vi "CALIBRATE 2016.vi"(0 "flow_slope_IN":dbl=51.35 format="%.2f", 1 "pressure_slope_IN":dbl=23.33 format="%.2f", 3 "DHT_Pressure Slope":dbl=1.5 format="%.2f", 4 "Descriptions":string[](array[string]), 5 "string_pot_slope_IN":dbl=1.5 format="%.2f", 6 "DHT_Pressure_Offset":dbl=1.5 format="%.2f", 7 "error in (no error)":errorcluster, 8 "Array in":refnum<k24>[](array[refnum]), 9 "Sensor Cluster":T2, 12 "Aux1_Slope In":dbl=1.5 format="%.2f", 13 "Aux3_ Slope In":dbl=1.5 format="%.2f", 16 "Aux2_Slope In":dbl=1.5 format="%.2f", 17 "Path":path=path "C:/Cascade/Data/Output Files") -> (14 "Array out":refnum<k24>[](array[refnum]), 15 "Sensor Cluster 2":T2, 19 "Output Slopes Cluster":T1={"DHT_Pressure Slope Out"=1.5, "DHT_Pressure_Offset Out"=1.5, "Aux1_Slope Out"=1.5, "Aux2_Slope Out"=1.5, "Aux3_ Slope Out"=1.5, "string_pot_slope_OUT"=1.5, "flow_slope_OUT"=51.35, "pressure_slope_OUT"=23.33} {"pressure_slope_OUT" format="%.2f"; "flow_slope_OUT" format="%.2f"; "string_pot_slope_OUT" format="%.2f"; "Aux3_ Slope Out" format="%.2f"; "Aux2_Slope Out" format="%.2f"; "Aux1_Slope Out" format="%.2f"; "DHT_Pressure_Offset Out" format="%.2f"; "DHT_Pressure Slope Out" format="%.2f"}, 20 "flow_slope_OUT":dbl=51.35 format="%.2f", 21 "pressure_slope_OUT":dbl=23.33 format="%.2f", 23 "Record Output Slopes to  Record File":path, 24 "Record Output Slopes for slopes.csv File":path, 25 "string_pot_slope_OUT":dbl=1.5 format="%.2f", 27 "error out":errorcluster)   [LabVIEW 2016]
uses:
  controls/MCC DAQ Readings.ctl
  C:/Program Files/National Instruments/LabVIEW 2016/vi.lib/ULx/ULx_LV.dll
  Program Files/National Instruments/LabVIEW 2016/vi.lib/ULx/ULx_LV.dll
  Kpro Globals.vi
panel:
  in  "Distance from APS Tip to transducer (ft)":dbl=5.2 format="%.2f"
  out "Aux3_ Slope Out":dbl=1.5 format="%.2f"
  out "Aux2_Slope Out":dbl=1.5 format="%.2f"
  out "Aux1_Slope Out":dbl=1.5 format="%.2f"
  out "DHT_Pressure_Offset Out":dbl=1.5 format="%.2f"
  out "DHT_Pressure Slope Out":dbl=1.5 format="%.2f"
  in  "all PFS":bool
  in  "Aux 3 Calibrate":bool
  in  "Aux 2 Calibrate":bool
  in  "Aux 1 Calibrate":bool
  in  "DHT":bool
  out "Loop Counter":i32
  in  "exit":bool
  in  "string_pot":bool
  in  "pressure":bool
  in  "flow":bool
  in  "start path":path=path "C:/"
  in  "all":bool
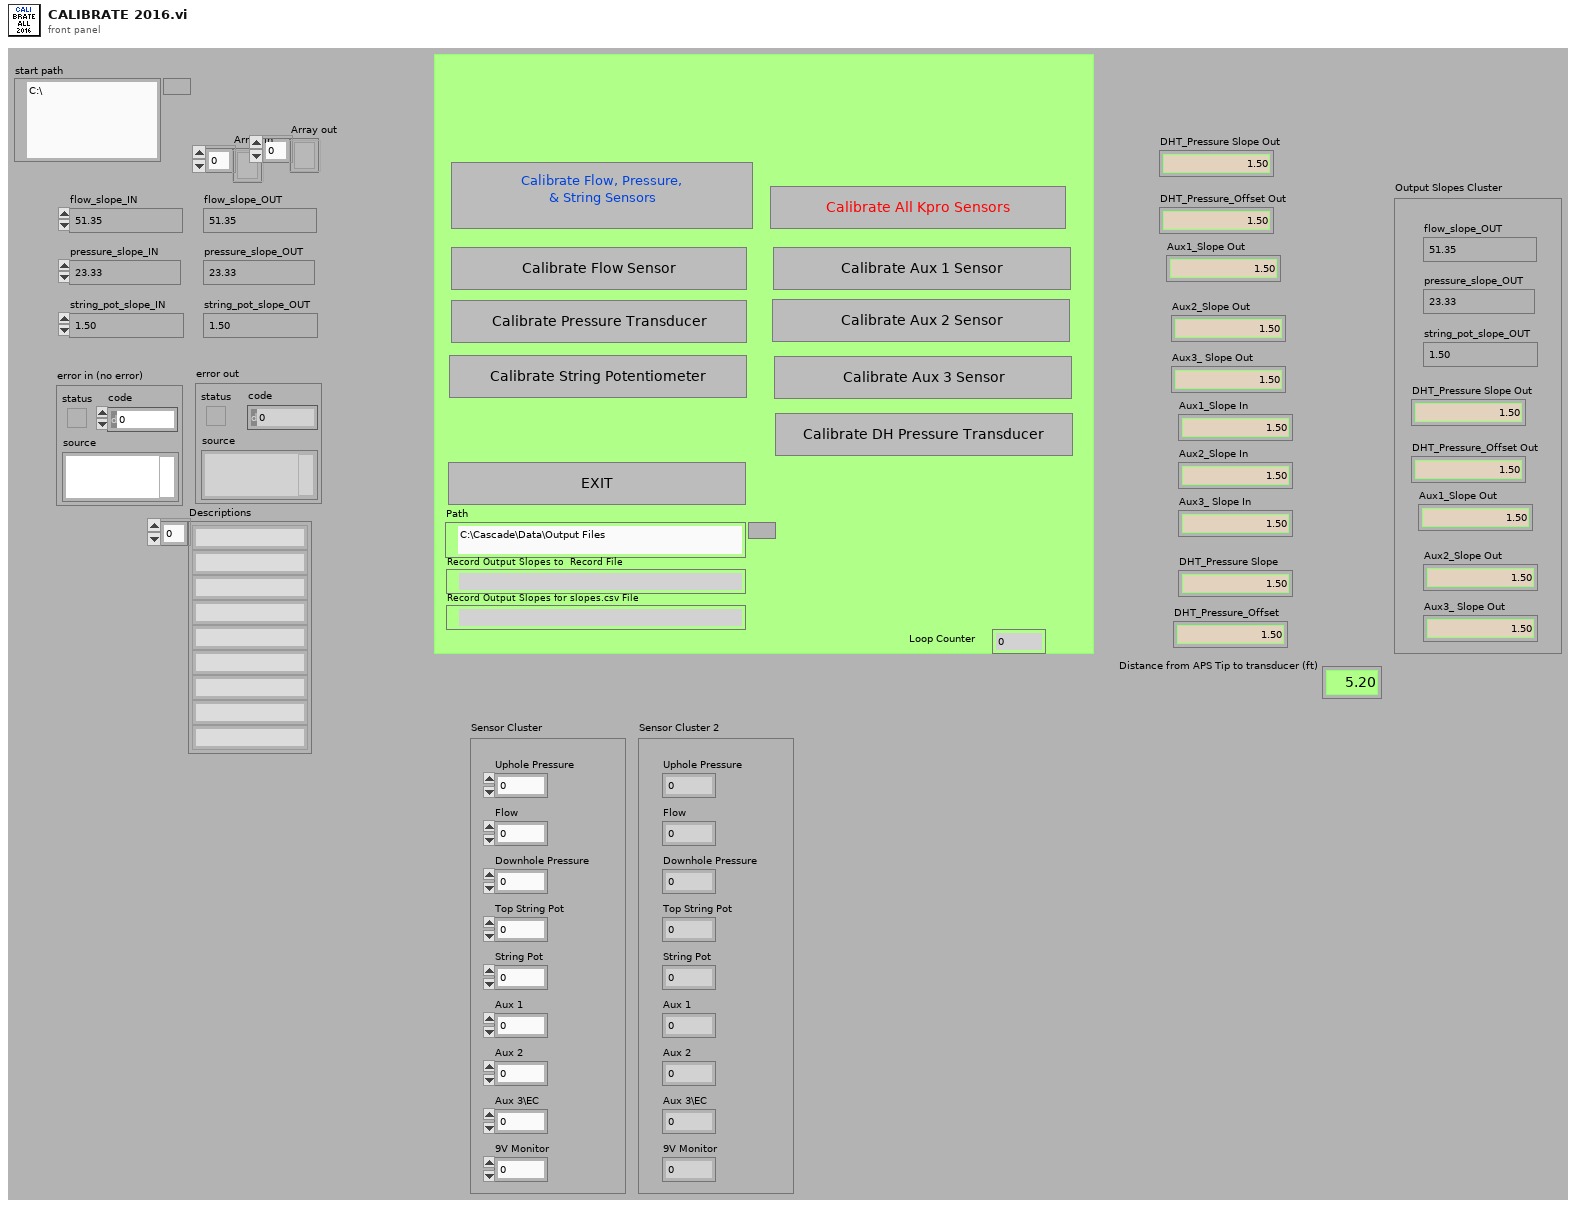
[diagram p1: front panel]
types:
  T1 = cluster{"DHT_Pressure Slope Out":dbl, "DHT_Pressure_Offset Out":dbl, "Aux1_Slope Out":dbl, "Aux2_Slope Out":dbl, "Aux3_ Slope Out":dbl, "string_pot_slope_OUT":dbl, "flow_slope_OUT":dbl, "pressure_slope_OUT":dbl}
  T2 = typedef "MCC DAQ Readings.ctl" = cluster{"Uphole Pressure":dbl, "Flow":dbl, "Downhole Pressure":dbl, "Top String Pot":dbl, "String Pot":dbl, "Aux 1":dbl, "Aux 2":dbl, "Aux 3\\EC":dbl, "9V Monitor":dbl}
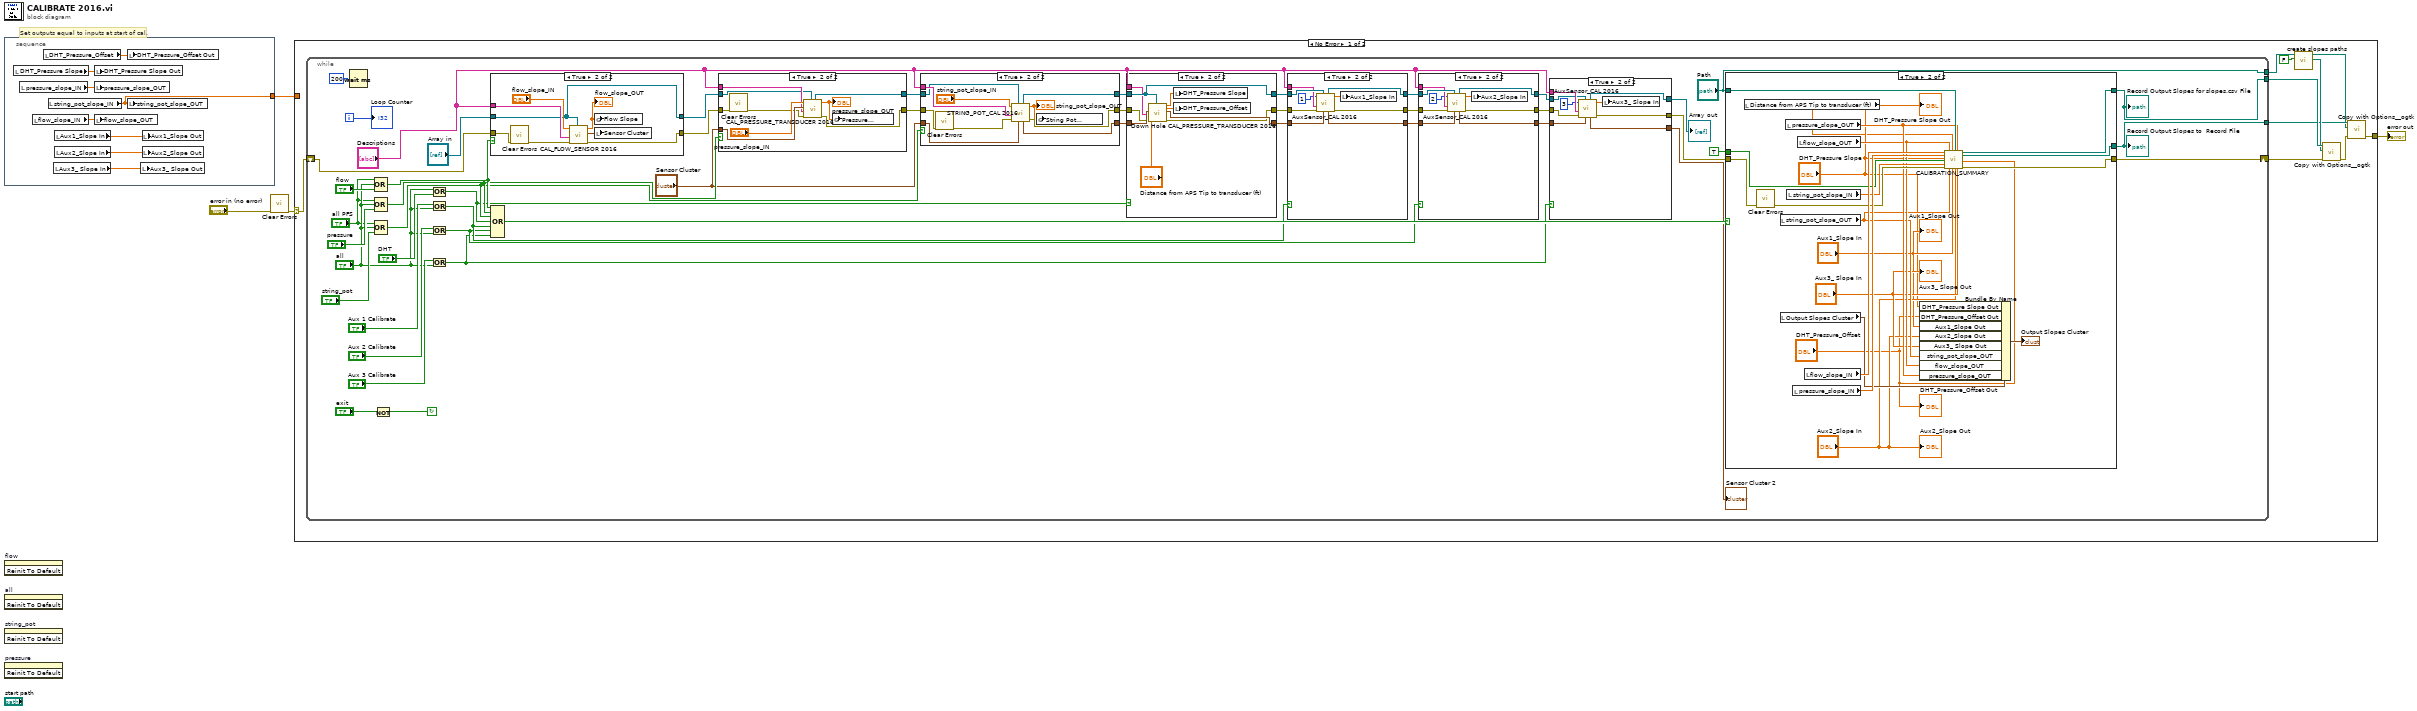
[diagram p0: block diagram]
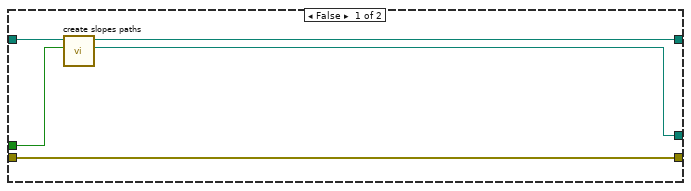
[diagram p6: hidden frame]
diagram:
  # "Set outputs equal to inputs at start of cal."
  n1 = stacked-sequence {
    tunnel: [w10] -> w2
    frame #0 {
      n2 = local read "DHT_Pressure Slope"() -> (w9:dbl)
      n3 = local read "pressure_slope_IN"() -> (w11:dbl)
      n4 = local read "flow_slope_IN"() -> (w12:dbl)
      n5 = local read "DHT_Pressure_Offset"() -> (w8:dbl)
      n6 = local read "string_pot_slope_IN"() -> (w10:dbl)
      n7 = local read "Aux3_ Slope In"() -> (w6:dbl)
      n8 = local read "Aux1_Slope In"() -> (w7:dbl)
      n9 = local read "Aux2_Slope In"() -> (w5:dbl)
      n10 = local write "DHT_Pressure Slope Out"(w9) -> ()
      n11 = local write "pressure_slope_OUT"(w11) -> ()
      n12 = local write "flow_slope_OUT"(w12) -> ()
      n13 = local write "DHT_Pressure_Offset Out"(w8) -> ()
      n14 = local write "string_pot_slope_OUT"(w10) -> ()
      n15 = local write "Aux3_ Slope Out"(w6) -> ()
      n16 = local write "Aux1_Slope Out"(w7) -> ()
      n17 = local write "Aux2_Slope Out"(w5) -> ()
    }
  }
  n18 = invoke on="flow" class="Bool" method="Reinit To Default"() -> ()  [unwired: 3 in, 3 out]
  n19 = invoke on="all" class="Bool" method="Reinit To Default"() -> ()  [unwired: 3 in, 3 out]
  n20 = invoke on="string_pot" class="Bool" method="Reinit To Default"() -> ()  [unwired: 3 in, 3 out]
  n21 = invoke on="pressure" class="Bool" method="Reinit To Default"() -> ()  [unwired: 3 in, 3 out]
  n22 = call <vilib>:"Clear Errors.vi"("error in (no error)"="error in (no error)") -> ("error out"=w1:errorcluster)  [unwired: 5 in, 1 out]
  n23 = case shown="No Error" w1 {
    selector: w1 -> [w22 w180]
    tunnel: [w13 w180] -> w3
    tunnel: w2 -> [_ _]
    frame No Error {
      n24 = while {
        shift-left: w22 -> [w68]
        shift-right: [w52] -> w14
        tunnel: ["Path"] -> w20
        tunnel: [w50] -> w19
        tunnel: [w49] -> w16
        i -> [w54]
        stop <- w71 continue-if-true
        n25 = Wait (ms)(milliseconds to wait=u32 200) -> ()  [unwired: 1 out]
        n26 = Compound Arithmetic op=OR("all PFS", "all", "flow") -> (w62:bool)
        n27 = Compound Arithmetic op=OR("all PFS", "all", "pressure") -> (w61:bool)
        n28 = Compound Arithmetic op=OR("all PFS", "all", "string_pot") -> (w60:bool)
        n29 = Not(x="exit") -> (.not. x?=w71:bool)
        n30 = Or(x="all", y="DHT") -> (x .or. y?=w47:bool)
        n31 = Or(x="Aux 1 Calibrate", y="all") -> (x .or. y?=w26:bool)
        n32 = Or(x="Aux 2 Calibrate", y="all") -> (x .or. y?=w25:bool)
        n33 = Or(x="Aux 3 Calibrate", y="all") -> (x .or. y?=w24:bool)
        n34 = case shown="True" w62 {
          tunnel: w68 -> [w171 w179]
          tunnel: [w171 w178] -> w65
          tunnel: "Descriptions" -> [_ w176]
          tunnel: "Array in" -> [w170 w175]
          tunnel: [w170 w175] -> w57
          frame False {
          }
          frame True {
            n35 = call <vilib>:"Clear Errors.vi"("error in (no error)"=w179) -> ("error out"=w173:errorcluster)  [unwired: 5 in, 1 out]
            n36 = call "CAL_FLOW_SENSOR 2016.vi"("Array in"=w175, "error in (no error)"=w173, "Descriptions"=w176, "flow_slope_IN"="flow_slope_IN") -> ("error out"=w178:errorcluster, "Sensor Cluster"=w174:T2, "flow_slope\nmL/min"=w172:dbl)  [unwired: 4 in, 1 out]
            "flow_slope_OUT" <- w172
            n37 = global write "Kpro Globals.vi" "Flow Slope"(w172) -> ()
            n38 = local write "Sensor Cluster"(w174) -> ()
          }
        }
        n39 = Compound Arithmetic op=OR(w62, w61, w60, w47, w26, w25, w24) -> (w59:bool)
        n40 = case shown="True" w61 {
          tunnel: [w160 w168] -> w66
          tunnel: w65 -> [w160 w169]
          tunnel: "Sensor Cluster" -> [_ w166]
          tunnel: "Descriptions" -> [_ w165]
          tunnel: w57 -> [w159 w164]
          tunnel: [w159 w163] -> w55
          frame False {
          }
          frame True {
            n41 = call <vilib>:"Clear Errors.vi"("error in (no error)"=w169) -> ("error out"=w162:errorcluster)  [unwired: 5 in, 1 out]
            n42 = call "CAL_PRESSURE_TRANSDUCER 2016.vi"("Array in"=w164, "error in (no error)"=w162, "Descriptions"=w165, "Sensor Cluster"=w166, "pressure_slope_IN"="pressure_slope_IN") -> ("error out"=w168:errorcluster, "pressure_slope_OUT"=w161:dbl, "Array out"=w163:refnum<k24>[])  [unwired: 3 in, 1 out]
            "pressure_slope_OUT" <- w161
            n43 = global write "Kpro Globals.vi" "Pressure \nSlope"(w161) -> ()
          }
        }
        n44 = case shown="True" w60 {
          tunnel: w66 -> [w148 w153]
          tunnel: [w148 w152] -> w44
          tunnel: "Descriptions" -> [_ w158]
          tunnel: "Sensor Cluster" -> [w147 w157]
          tunnel: w55 -> [w146 w156]
          tunnel: [w146 w155] -> w46
          tunnel: [w147 w151] -> w45
          frame False {
          }
          frame True {
            n45 = call <vilib>:"Clear Errors.vi"("error in (no error)"=w153) -> ("error out"=w150:errorcluster)  [unwired: 5 in, 1 out]
            n46 = call "STRING_POT_CAL 2016.vi"("Sensor Cluster"=w157, "Array in"=w156, "error in (no error)"=w150, "Descriptions"=w158, "string_pot_slope_IN"="string_pot_slope_IN") -> ("error out"=w152:errorcluster, "string_pot_slope_OUT"=w149:dbl, "Sensor Cluster 2"=w151:T2, "Array out"=w155:refnum<k24>[])  [unwired: 3 in]
            "string_pot_slope_OUT" <- w149
            n47 = global write "Kpro Globals.vi" "String Pot \nSlope"(w149) -> ()
          }
        }
        n48 = case shown="True" w47 {
          tunnel: w46 -> [w109 w119]
          tunnel: w45 -> [w110 w118]
          tunnel: [w109 w119] -> w39
          tunnel: [w110 w117] -> w31
          tunnel: "Descriptions" -> [_ w116]
          tunnel: w44 -> [w108 w115]
          tunnel: [w108 w114] -> w34
          frame False {
          }
          frame True {
            n49 = call "Down Hole CAL_PRESSURE_TRANSDUCER 2016.vi"("Distance from APS Tip to transducer (ft)"="Distance from APS Tip to transducer (ft)", "Sensor Cluster"=w118, "Descriptions"=w116, "error in (no error)"=w115, "Array in"=w119) -> ("Pressure\nSlope (psi/V)"=w113:dbl, "Pressure\nOffset (psi)"=w112:dbl, "Sensor Cluster 2"=w117:T2, "error out"=w114:errorcluster)  [unwired: 7 in, 4 out]
            n50 = local write "DHT_Pressure Slope"(w113) -> ()
            n51 = local write "DHT_Pressure_Offset"(w112) -> ()
          }
        }
        n52 = case shown="True" w26 {
          tunnel: [w98 w106] -> w38
          tunnel: w39 -> [w98 w107]
          tunnel: w34 -> [w97 w103]
          tunnel: [w97 w101] -> w36
          tunnel: w31 -> [w96 w102]
          tunnel: [w96 w104] -> w30
          tunnel: "Descriptions" -> [_ w105]
          frame False {
          }
          frame True {
            n53 = call "AuxSensor_CAL 2016.vi"("Sensor Cluster"=w102, "Array in"=w107, "error in (no error)"=w103, "Descriptions"=w105, "Aux Sensor"=1) -> ("error out"=w101:errorcluster, "Aux Sensor\nSlope (unit/V)"=w99:dbl, "Sensor Cluster 2"=w104:T2, "Array out"=w106:refnum<k24>[])  [unwired: 2 in, 1 out]
            n54 = local write "Aux1_Slope In"(w99) -> ()
          }
        }
        n55 = case shown="True" w25 {
          tunnel: [w86 w90] -> w37
          tunnel: w38 -> [w86 w91]
          tunnel: w36 -> [w85 w95]
          tunnel: [w85 w94] -> w35
          tunnel: w30 -> [w84 w93]
          tunnel: [w84 w92] -> w29
          tunnel: "Descriptions" -> [_ w89]
          frame False {
          }
          frame True {
            n56 = call "AuxSensor_CAL 2016.vi"("Sensor Cluster"=w93, "Array in"=w91, "error in (no error)"=w95, "Descriptions"=w89, "Aux Sensor"=2) -> ("error out"=w94:errorcluster, "Aux Sensor\nSlope (unit/V)"=w87:dbl, "Sensor Cluster 2"=w92:T2, "Array out"=w90:refnum<k24>[])  [unwired: 2 in, 1 out]
            n57 = local write "Aux2_Slope In"(w87) -> ()
          }
        }
        n58 = case shown="True" w24 {
          tunnel: [w74 w79] -> w32
          tunnel: w37 -> [w74 w80]
          tunnel: w35 -> [w73 w83]
          tunnel: [w73 w82] -> w33
          tunnel: w29 -> [w72 w78]
          tunnel: [w72 w77] -> w28
          tunnel: "Descriptions" -> [_ w81]
          frame False {
          }
          frame True {
            n59 = call "AuxSensor_CAL 2016.vi"("Sensor Cluster"=w78, "Array in"=w80, "error in (no error)"=w83, "Descriptions"=w81, "Aux Sensor"=3) -> ("error out"=w82:errorcluster, "Aux Sensor\nSlope (unit/V)"=w75:dbl, "Sensor Cluster 2"=w77:T2, "Array out"=w79:refnum<k24>[])  [unwired: 2 in, 1 out]
            n60 = local write "Aux3_ Slope In"(w75) -> ()
          }
        }
        "Array out" <- w32
        "Sensor Cluster 2" <- w28
        n61 = case shown="True" w59 {
          tunnel: w33 -> [w124 w145]
          tunnel: [w124 w144] -> w52
          tunnel: "Path" -> [w123 w139]
          tunnel: [w121 w138] -> w50
          tunnel: [w122 w137] -> w49
          tunnel: TRUE ("Strip Path") -> [w120 w136]
          frame False {
            n62 = call "create slopes paths.vi"("Strip Path"=w120, "Path"=w123) -> ("Record Output Slopes for slopes.csv File"=w122:path, "Record Output Slopes to  Record File"=w121:path)  [unwired: 8 in]
          }
          frame True {
            n63 = local read "Distance from APS Tip to transducer (ft)"() -> (w125:dbl)
            n64 = call <vilib>:"Clear Errors.vi"("error in (no error)"=w145) -> ("error out"=w140:errorcluster)  [unwired: 5 in, 1 out]
            n65 = local read "string_pot_slope_OUT"() -> (w131:dbl)
            n66 = local read "Output Slopes Cluster"() -> (w135:T1)
            n67 = local read "pressure_slope_OUT"() -> (w133:dbl)
            n68 = local read "string_pot_slope_IN"() -> (w141:dbl)
            n69 = local read "pressure_slope_IN"() -> (w142:dbl)
            n70 = local read "flow_slope_OUT"() -> (w132:dbl)
            n71 = local read "flow_slope_IN"() -> (w143:dbl)
            n72 = Bundle By Name(cluster=w135, "DHT_Pressure Slope Out"="DHT_Pressure Slope", "DHT_Pressure_Offset Out"="DHT_Pressure_Offset", "Aux1_Slope Out"="Aux1_Slope In", "Aux2_Slope Out"="Aux2_Slope In", "Aux3_ Slope Out"="Aux3_ Slope In", "string_pot_slope_OUT"=w131, "flow_slope_OUT"=w132, "pressure_slope_OUT"=w133) -> (→"Output Slopes Cluster":T1)
            n73 = call "CALIBRATION_SUMMARY.vi"("flow_slope_IN"=w143, "pressure_slope_IN"=w142, "DHT_Pressure_In"="DHT_Pressure Slope", "Strip Path"=w136, "string_pot_slope_IN"=w141, "error in (no error)"=w140, "flow_slope_OUT"=w132, "string_pot_slope_OUT"=w131, "Distance from APS Tip to transducer (ft)"=w125, "Aux1_In"="Aux1_Slope In", "Path"=w139, "Aux2_In"="Aux2_Slope In", "pressure_slope_OUT"=w133, "Aux3_In"="Aux3_ Slope In", "DHT_Pressure_In Offset"="DHT_Pressure_Offset") -> ("Record Output Slopes for slopes.csv File"=w138:path, "Record Output Slopes to  Record File"=w137:path, "error out"=w144:errorcluster)  [unwired: 2 in]
            "DHT_Pressure Slope Out" <- "DHT_Pressure Slope"
            "DHT_Pressure_Offset Out" <- "DHT_Pressure_Offset"
            "Aux1_Slope Out" <- "Aux1_Slope In"
            "Aux2_Slope Out" <- "Aux2_Slope In"
            "Aux3_ Slope Out" <- "Aux3_ Slope In"
          }
        }
        "Record Output Slopes for slopes.csv File" <- w50
        "Record Output Slopes to  Record File" <- w49
        "Loop Counter" <- w54
      }
      n74 = call "create slopes paths.vi"("Strip Path"=FALSE, "Path"=w20) -> ("Record Output Slopes for slopes.csv File"=w18:path, "Record Output Slopes to  Record File"=w15:path)  [unwired: 8 in]
      n75 = call <userlib>:"Copy with Options__ogtk.vi"("error in (no error)"=w14, "target path"=w18, "source path"=w19) -> ("error out"=w17:errorcluster)  [unwired: 7 in, 1 out]
      n76 = call <userlib>:"Copy with Options__ogtk.vi"("error in (no error)"=w17, "target path"=w15, "source path"=w16) -> ("error out"=w13:errorcluster)  [unwired: 7 in, 1 out]
    }
    frame Error {
    }
  }
  "error out" <- w3
